vi "DQMH System Message - Remove from Run-Time Menu.vi"(11 "Main VI Reference":refnum<vi>) -> (1 "Payload":variant, 2 "Identifier":string="Add to Run-Time Menu", 5 "Source":T1)   [LabVIEW 2022 SP3, in "hse-dqmh.lvlib"]
doc: "____\nHAMPEL SOFTWARE ENGINEERING v3.8.0 (2023-12-18 14:41)"
uses:
  hse-dqmh.lvlib
  Controls/System Message Source.ctl
  Controls/System Message Framework Identifiers.ctl
  Controls/System Message - Remove from Run-Time Menu - Argument--cluster.ctl
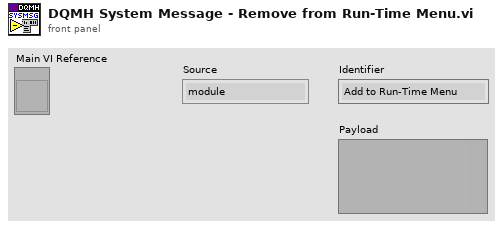
[diagram p1: front panel]
types:
  T1 = typedef "hse-dqmh.lvlib/System Message Source.ctl" = enum16{"module", "application", "network"}
  T2 = typedef "hse-dqmh.lvlib/System Message - Remove from Run-Time Menu - Argument--cluster.ctl" = cluster{"Module Disk Path":path}
  T3 = typedef "hse-dqmh.lvlib/System Message Framework Identifiers.ctl" = enum16{"Add to Run-Time Menu", "Ready for Display", "Removed from Subpanel", "Remove from Run-Time Menu"}
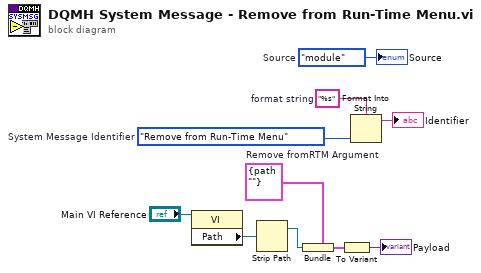
[diagram p0: block diagram]
diagram:
  w1 = T2 {"Module Disk Path"=path ""}  # Remove fromRTM Argument
  w6 = "%s"  # format string
  w8 = System_Message_Framework_Identifiers."Remove from Run-Time Menu"  # System Message Identifier
  w10 = System_Message_Source."module"  # Source
  n1 = property class="VI"(reference="Main VI Reference") -> ("Path"=w4:path)  [unwired: 1 in, 2 out]
  n2 = Strip Path(path=w4) -> (stripped path=w2:path)  [unwired: 1 out]
  n3 = Bundle(cluster=w1, "Module Disk Path"=w2) -> (w5:T2)
  n4 = To Variant(anything=w5) -> (Variant=→"Payload":variant)
  n5 = Format Into String(format string=w6, w8) -> (resulting string=→"Identifier":string)  [unwired: 2 in, 1 out]
  "Source" <- w10
